vi "main.vi"() -> ()   [LabVIEW 2012]
doc: "Use this template to build a user interface event handler design pattern. Use this pattern for dialog boxes and other user interfaces. You also can create and execute user-defined events that the VI can handle the same way as user interface events."
uses:
  <vilib>/Utility/file.llb/Read From Spreadsheet File (DBL).vi
  <vilib>/Analysis/baseanly.llb/Mean (DBL).vi
  <vilib>/vision/NI_Vision_Development_Module.lvlib
  <vilib>/Analysis/NI_AALBase.lvlib
panel:
  in  "timetrace":i32=10
  in  "export image":bool
  in  "intervals":i32=10
  out "Histogram":T1(graph)
  out "Total":dbl format="%#_4p"
  out "Signal":dbl format="%0.2f"
  out "Background":dbl format="%0.2f"
  out "Timetrace":dbl[](graph)
  in  "Tab Control":enum32{"Image", "Raw data"}(tab)
  out "Image":T2(plugin-control)
  out "Intensity Graph":dbl[][](graph)
  in  "Read File1":bool
  in  "stop":bool
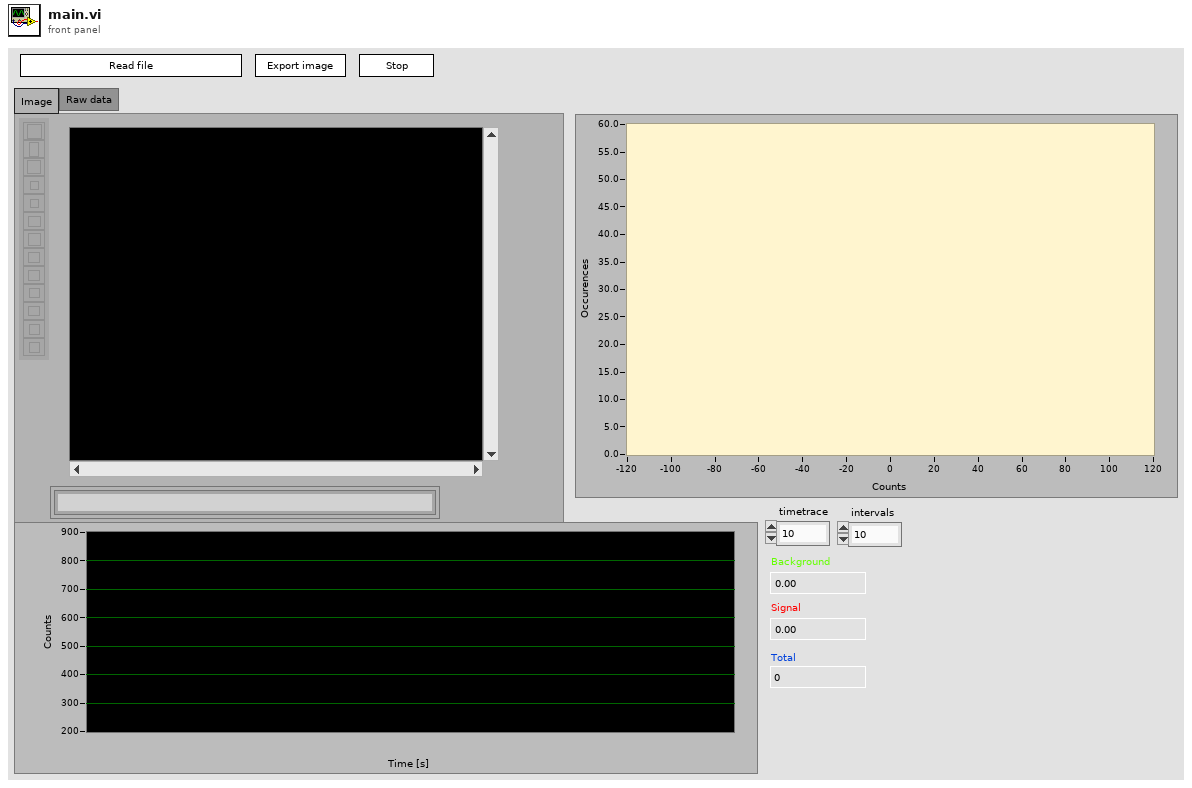
[diagram p1: front panel]
types:
  T1 = cluster{"X Values":dbl[], "Histogram: h(x)":i32[]}[]
  T2 = typedef "IMAQ Image.ctl" = refnum<image>
  T3 = typedef "Image Type" = u32
  T4 = typedef "Image Unit" = enum32{"Undefined", "Angström", "Micrometer", "Millimeter", "Centimeter", "Meter", "Kilometer", "Microinch", "Inch", "Feet", "Nautical miles", "Standard miles", "Steps"}
  T5 = typedef "Simple Grid Descriptor" = cluster{"X Step":sgl, "Y Step":sgl, "Unit":T4}
  T6 = cluster{"Bounding Rectangle":cluster{"Left":i32, "Top":i32, "Right":i32, "Bottom":i32}, string}[]
  T7 = cluster{"X Values":dbl[], "Histogram: h(x)":i32[]}
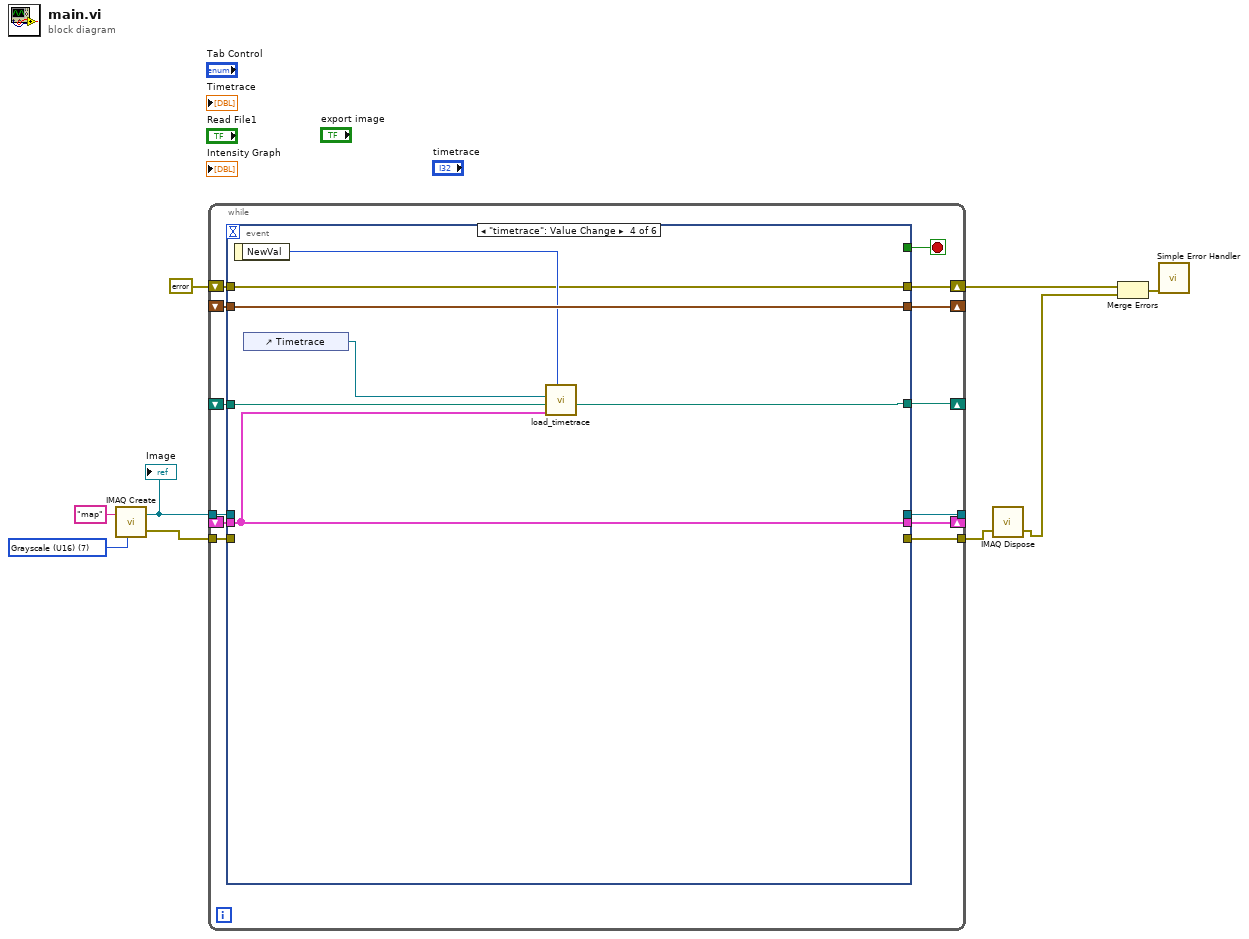
[diagram p0: block diagram]
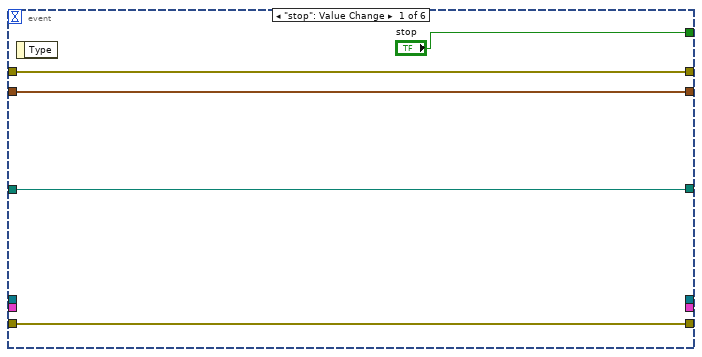
[diagram p2: hidden frame]
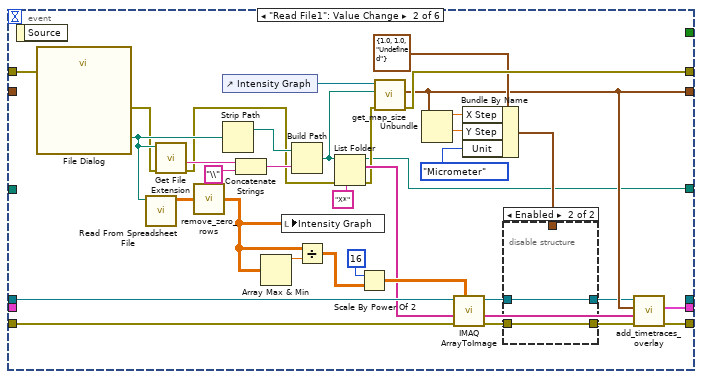
[diagram p3: hidden frame]
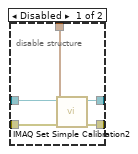
[diagram p4: hidden frame]
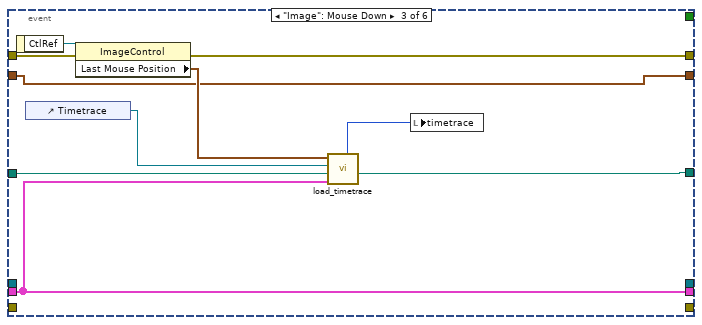
[diagram p5: hidden frame]
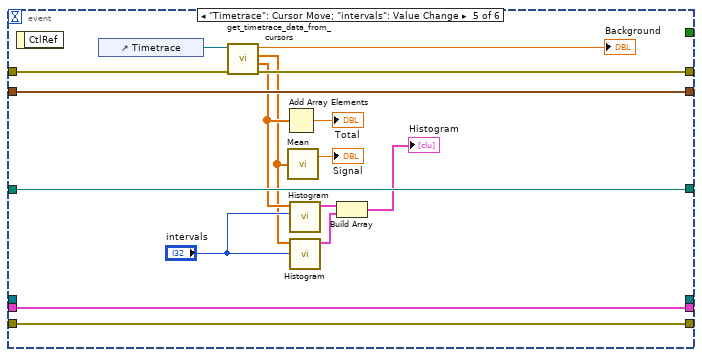
[diagram p6: hidden frame]
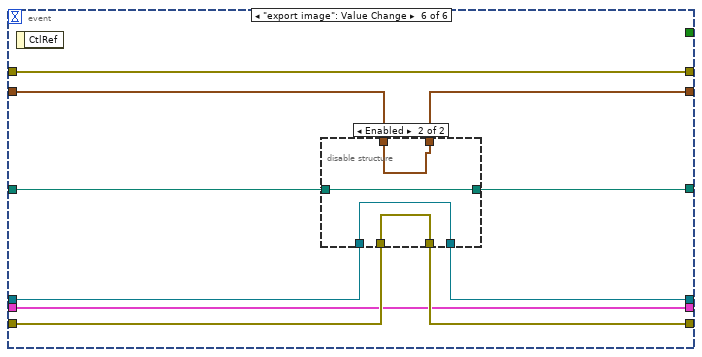
[diagram p7: hidden frame]
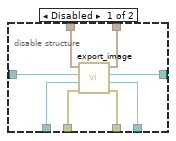
[diagram p8: hidden frame]
diagram:
  w7 = T3 7 items=["Grayscale (U8)", "Grayscale (I16)", "Grayscale (SGL)", "Complex (CSG)", "RGB (U32)", "HSL (U32)", "RGB (U64)", "Grayscale (U16)"] ("Image Type")
  n1 = call "IMAQ Create"("Image Name"="map", "Image Type"=w7) -> ("New Image"=w5:T2, "error out"=w6:errorcluster)  [unwired: 3 in]
  "Image" <- w5
  n2 = while {
    shift-right: [w20] -> w3
    shift-left: errorcluster {"status"=FALSE, "code"=0, "source"=""} ("error in") -> [w21]
    tunnel: w5 -> [w19]
    tunnel: w6 -> [w18]
    tunnel: [w17] -> _
    tunnel: [w16] -> w4
    shift-right: [w15] -> _
    shift-left: _ -> [w14]
    shift-right: [w13] -> _
    shift-left: _ -> [w12]
    shift-right: [w11] -> _
    shift-left: _ -> [w10]
    stop <- w22 stop-if-true
    n3 = event shown="[3] \"timetrace\": Value Change" {
      selector: _ -> [_ _ _ _ _ _]
      dyn-events: _ -> [_ _ _ _ _ _]
      timeout: _ -> [_ _ _ _ _ _]
      tunnel: ["stop" _ _ _ _ _] -> w22
      tunnel: w21 -> [w26 w62 w77 w79 w96 w107]
      tunnel: [w26 w53 w71 w79 w94 w107] -> w20
      tunnel: w19 -> [_ w51 _ _ _ w103]
      tunnel: w18 -> [w25 w50 _ _ w98 w109]
      tunnel: [_ _ _ _ _ w104] -> w17
      tunnel: [w25 w35 _ _ w98 w108] -> w16
      tunnel: [w24 w40 w72 w81 w97 w105] -> w15
      tunnel: w14 -> [w24 _ w72 w81 w97 w101]
      tunnel: [_ w31 w74 w83 w99 w102] -> w13
      tunnel: w12 -> [_ _ w74 w83 w99 w102]
      tunnel: [w23 w30 w73 w82 w95 w106] -> w11
      tunnel: w10 -> [w23 _ w73 w82 w95 w110]
      event "stop": Value Change {
        n4 = event-data() -> ()  [unwired: 1 in, 1 out]
      }
      event "Read File1": Value Change {
        n5 = event-data() -> ()  [unwired: 1 in, 1 out]
        n6 = call "File Dialog"("error in"=w62) -> ("selected path"=w60:path, "error out"=w52:errorcluster)  [unwired: 11 in, 2 out]
        n7 = call-poly <vilib>:"Read From Spreadsheet File.vi"("file path (dialog if empty)"=w60) -> ("all rows"=w29:dbl[][])  [unwired: 6 in, 4 out]
        n8 = call <vilib>:"Get File Extension.vi"("error in (no error)"=w52, "file"=w60) -> ("error out"=w33:errorcluster, "filename without extension"=w59:string)  [unwired: 6 in, 2 out]
        n9 = call "remove_zero_rows.vi"("all rows in"=w29) -> ("all rows out"=w28:dbl[][])
        n10 = control-ref of="Intensity Graph"() -> (w54:refnum<vi>)
        n11 = Strip Path(path=w60) -> (stripped path=w61:path)  [unwired: 1 out]
        n12 = Concatenate Strings(w59, "\\" ("string")) -> (w58:string)
        n13 = Array Max & Min(array=w28) -> (max value=w49:dbl)  [unwired: 3 out]
        n14 = local write "Intensity Graph"(w28) -> ()
        n15 = Build Path(base path=w61, name or relative path=w58) -> (appended path=w55:path)
        n16 = Divide(x=w28, y=w49) -> (x/y=w48:dbl[][])
        n17 = List Folder(path=w55, pattern="X*", error in=w33) -> (path out=w30:path, filenames=w34:string[], error out=w32:errorcluster)  [unwired: 1 in, 1 out]
        n18 = Scale By Power Of 2(n=i16 16, x=w48) -> (x*2^n=w46:dbl[][])
        n19 = call "get_map_size.vi"("error in (no error)"=w32, "appended path"=w55, "IntensityGraph in"=w54) -> ("error out"=w53:errorcluster, "map size"=w40:cluster{dbl, dbl, dbl, dbl})  [unwired: 7 in]
        n20 = Unbundle(w40) -> (w44:dbl, w43:dbl)  [unwired: 2 out]
        n21 = call "IMAQ ArrayToImage"("Image Pixels (U16)"=w46, "error in (no error)"=w50, "Image"=w51) -> ("error out"=w38:errorcluster, "Image Out"=w39:T2)  [unwired: 7 in]
        n22 = Bundle By Name(cluster=T5 {"X Step"=1.0, "Y Step"=1.0, "Unit"=enum."Undefined"} ("Pixel Distances"), "X Step"=w44, "Y Step"=w43, "Unit"=Image_Unit."Micrometer") -> (w41:T5)
        n23 = disable-structure shown="Enabled" {
          disable-tunnel: w41 -> [w67 _]
          disable-tunnel: w39 -> [w66 w69]
          disable-tunnel: w38 -> [w65 w68]
          disable-tunnel: [w64 w69] -> w37
          disable-tunnel: [w63 w68] -> w36
          frame Disabled {
            n24 = call "IMAQ Set Simple Calibration2"("error in (no error)"=w65, "Pixel Distances"=w67, "Image"=w66) -> ("error out"=w63:errorcluster, "Calibration Template Image"=w64:T2)  [unwired: 7 in]
          }
          frame Enabled {
          }
        }
        n25 = call "add_timetraces_overlay.vi"("error in (no error)"=w36, "filenames"=w34, "map size"=w40, "Refnum in"=w37) -> ("error out"=w35:errorcluster, "Timetraces"=w31:T6)  [unwired: 5 in, 1 out]
      }
      event "Image": Mouse Down {
        n26 = event-data() -> ("CtlRef"=w78:refnum<vi>)  [unwired: 1 in]
        n27 = control-ref of="Timetrace"() -> (w75:refnum<vi>)
        n28 = property on="Property Node" class="ImageControl"(reference=w78, error in=w77) -> (error out=w71:errorcluster, "Last Mouse Position"=w76:cluster{"X":i32, "Y":i32})  [unwired: 1 out]
        n29 = call "load_timetrace.vi"("Timetraces"=w74, "path in"=w73, "WaveformGraph in"=w75, "Last Mouse Position"=w76) -> ("index"=w70:i32)  [unwired: 7 in]
        n30 = local write "timetrace"(w70) -> ()
      }
      event "timetrace": Value Change {
        n31 = event-data() -> ("NewVal"=w80:i32)  [unwired: 1 in]
        n32 = control-ref of="Timetrace"() -> (w84:refnum<vi>)
        n33 = call "load_timetrace.vi"("index"=w80, "Timetraces"=w83, "path in"=w82, "WaveformGraph in"=w84) -> ()  [unwired: 7 in, 1 out]
      }
      event "Timetrace": Cursor Move; "intervals": Value Change {
        n34 = event-data() -> ()  [unwired: 1 in, 1 out]
        n35 = control-ref of="Timetrace"() -> (w100:refnum<vi>)
        n36 = call "get_timetrace_data_from_cursors.vi"("error in (no error)"=w96, "WaveformGraph in"=w100) -> ("error out"=w94:errorcluster, "Array 2"=w91:dbl[], "Array"=w85:dbl[], "mean"=→"Background":dbl)  [unwired: 6 in]
        n37 = Add Array Elements(numeric array=w91) -> (sum=→"Total":dbl)
        n38 = call-poly <vilib>:"Mean.vi"("X"=w85) -> ("mean"=→"Signal":dbl)  [unwired: 1 out]
        n39 = call <vilib>:"Histogram.vi"("intervals"="intervals", "X"=w91) -> ("Histogram Graph"=w89:T7)  [unwired: 6 in, 3 out]
        n40 = call <vilib>:"Histogram.vi"("intervals"="intervals", "X"=w85) -> ("Histogram Graph"=w88:T7)  [unwired: 6 in, 3 out]
        n41 = Build Array(w89, w88) -> (→"Histogram":T1)
      }
      event "export image": Value Change {
        n42 = event-data() -> ()  [unwired: 1 in, 1 out]
        n43 = disable-structure shown="Enabled" {
          disable-tunnel: w110 -> [w118 w121]
          disable-tunnel: w109 -> [w117 w119]
          disable-tunnel: [w116 w119] -> w108
          disable-tunnel: [w115 w121] -> w106
          disable-tunnel: [w114 w122] -> w105
          disable-tunnel: [w113 w120] -> w104
          disable-tunnel: w103 -> [w112 w120]
          disable-tunnel: w101 -> [w111 w122]
          frame Disabled {
            n44 = call "export_image.vi"("error in (no error)"=w117, "Refnum in"=w112, "path in"=w118, "map size in"=w111) -> ("error out"=w116:errorcluster, "Refnum out"=w113:T2, "path out"=w115:path, "map size out"=w114:cluster{dbl, dbl, dbl, dbl})  [unwired: 4 in]
          }
          frame Enabled {
          }
        }
      }
    }
  }
  n45 = call "IMAQ Dispose"("error in (no error)"=w4) -> ("error out"=w2:errorcluster)  [unwired: 5 in]
  n46 = Merge Errors(w3, w2) -> (w1:errorcluster)
  n47 = call <vilib>:"Simple Error Handler.vi"("error in (no error)"=w1) -> ()  [unwired: 4 in, 5 out]
